vi "Terminate.vi"(8 "error in (no error)":errorcluster, 11 "UnitTestEngine in":refnum<class "UnitTestEngine.lvclass">) -> (0 "error out":errorcluster, 3 "UnitTestEngine out":refnum<class "UnitTestEngine.lvclass">)   [LabVIEW 2019, in "UnitTestEngine.lvlib" / "UnitTestEngine.lvclass"]
uses:
  UnitTestEngine.lvclass
  TestEngine/TestEngine/TestEngine.lvclass
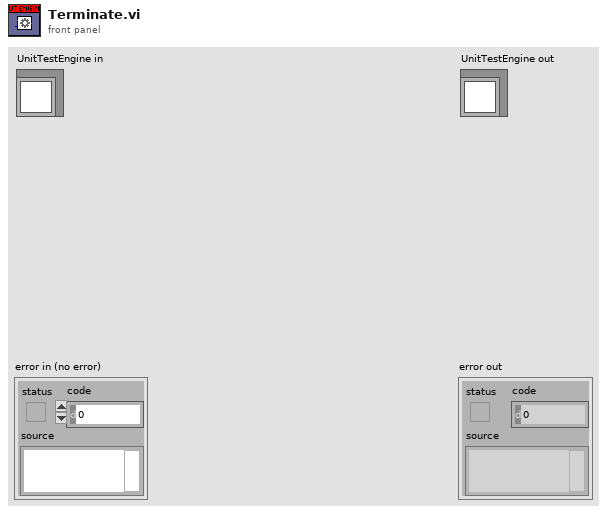
[diagram p1: front panel]
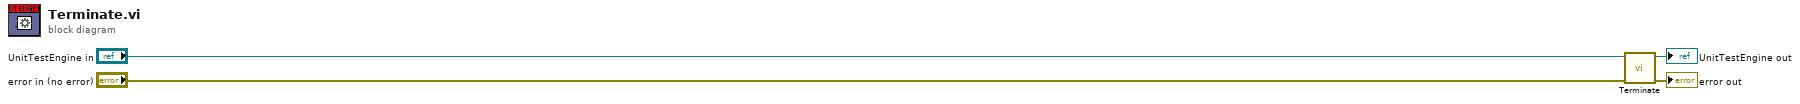
[diagram p0: block diagram]
diagram:
  n1 = call-parent "Terminate.vi"("error in (no error)"="error in (no error)", "TestEngine in"="UnitTestEngine in") -> ("error out"=→"error out":errorcluster, "TestEngine out"=→"UnitTestEngine out":refnum<class "UnitTestEngine.lvclass">)  [unwired: 8 in]
